vi "Close.vi"(8 "error in (no error)":errorcluster, 11 "Simple Device in":refnum<class "Simple Device.lvclass">) -> (0 "error out":errorcluster, 3 "Simple Device out":refnum<class "Simple Device.lvclass">)   [LabVIEW 2021, in "Simple Device.lvclass"]
uses:
  Simple Device.lvclass
  Simple Device.lvclass/Simple Device.ctl
  TALOS/TALOS_PPL.lvlibp
  Libraries/Virtual Device Simulator/DeviceSim.lvlibp/DeviceReference/Simple  Virtual Device.lvclass
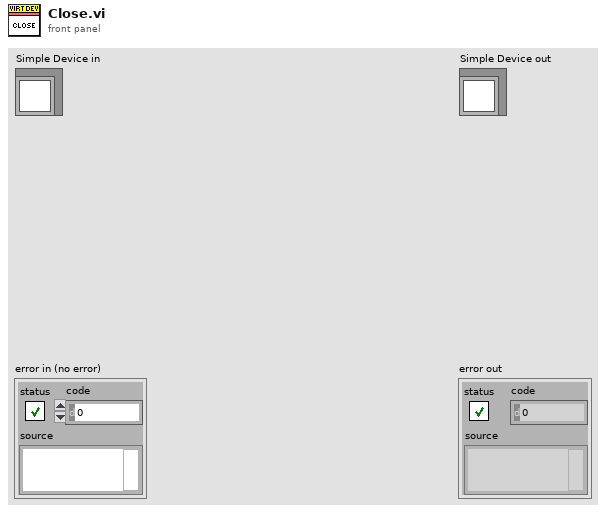
[diagram p1: front panel]
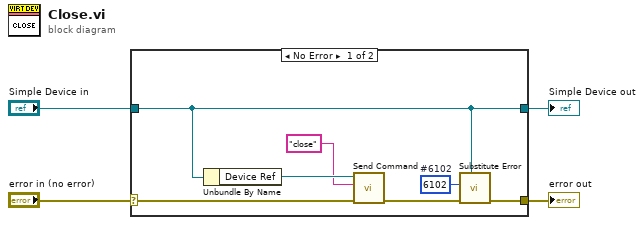
[diagram p0: block diagram]
diagram:
  n1 = case shown="No Error" "error in (no error)" {
    selector: "error in (no error)" -> [w6 w13]
    tunnel: [w11 w13] -> w3
    tunnel: [w10 w12] -> w1
    tunnel: "Simple Device in" -> [w10 w12]
    frame No Error {
      w9 = 6102  # #6102
      n2 = Unbundle By Name(w10) -> ("Device Ref"=w8:refnum<data-value>)
      n3 = call "Send Command.vi"("error in (no error)"=w6, "Command"="close", "Device Ref in"=w8) -> ("error out"=w5:errorcluster)  [unwired: 6 in, 2 out]
      n4 = call "Substitute Error.vi"("LabVIEW Object"=w10, "error in (no error)"=w5, "Error Code"=w9) -> ("error out"=w11:errorcluster)  [unwired: 8 in]
    }
    frame Error {
    }
  }
  "error out" <- w3
  "Simple Device out" <- w1
